vi "Software name constant.vi"() -> (0 "Software name constant":string)   [LabVIEW 2018]
doc: "Get the software name constant here. Keep it short if possible (3 words or less, under 30 characters).\n\nNote that this is the SOFTWARE name, not the STATION name, as the same software might run on multiple stations!"
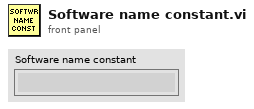
[diagram p1: front panel]
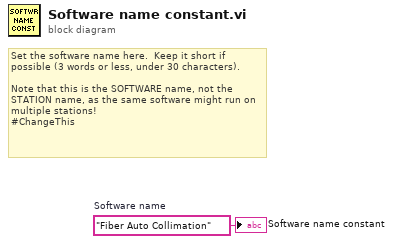
[diagram p0: block diagram]
diagram:
  w1 = "Fiber Auto Collimation"  # Software name
  # "Set the software name here.  Keep it short if possible (3 words or less, under 30 characters).\n\nNote that this is the SOFTWARE name, not the STATION name, as the same software might run on multiple stations!\n#ChangeThis"
  "Software name constant" <- w1
